vi "GV PMT sim.vi"() -> ()   [LabVIEW 2017]
panel:
  out "PMT sim":bool
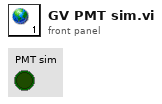
[diagram p1: front panel]
diagram:
